vi "vSwap.vi"   [LabVIEW 2020]
doc: "SWAP Gate (should be paired with an other qubit)\n\nExchanges the states of two qubits. \n\nMatrix: [[ 1, 0, 0, 0], [ 0, 0, 1, 0], [ 0, 1, 0, 0], [ 0, 0, 0, 1]]"
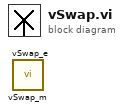
[diagram p0: block diagram]
diagram:
  n1 = call "vSwap_m.vi"() -> ()  [unwired: 14 in, 2 out]
  n2 = call "vSwap_e.vi"() -> ()  [unwired: 14 in, 2 out]
